vi "calc global ODMR and norm for stack (MW on-off).vi"(8 "Height":i64(slide)=1200 min=0 max=1200 step=4 scale=0.0..1200.0, 9 "Width":i64(slide)=1920 min=0 max=1920 step=4 scale=0.0..1920.0, 10 "sweep #":i32, 11 "img data stack":dbl[][](array[numeric])) -> (3 "normed spectrum":dbl[](array[numeric]))   [LabVIEW 2019]
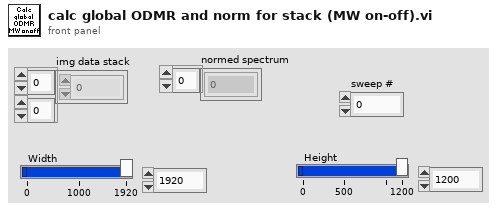
[diagram p1: front panel]
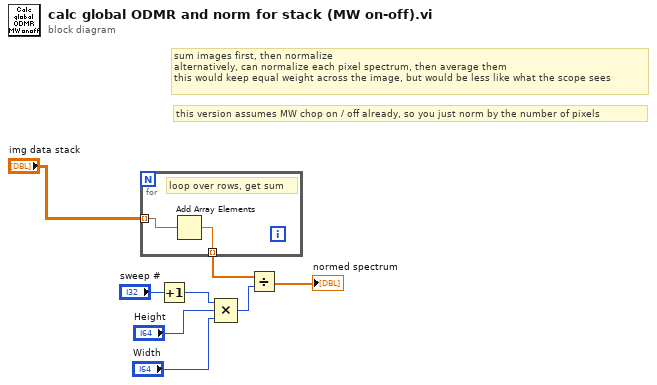
[diagram p0: block diagram]
diagram:
  # "this version assumes MW chop on / off already, so you just norm by the number of pixels"
  # "sum images first, then normalize\nalternatively, can normalize each pixel spectrum, then average them\nthis would keep equal weight across the image, but would be less like what the scope sees"
  n1 = for {
    tunnel: "img data stack" -> [w10] mode=indexing
    tunnel: [w9] -> w6 mode=indexing
    # "loop over rows, get sum"
    n2 = Add Array Elements(numeric array=w10) -> (sum=w9:dbl)
  }
  n3 = Increment(x="sweep #") -> (x+1=w1:i32)
  n4 = Compound Arithmetic op=MULTIPLY(w1, "Height", "Width") -> (w5:i64)
  n5 = Divide(x=w6, y=w5) -> (x/y=→"normed spectrum":dbl[])
